vi "MSScript VI Example.vi"() -> ()   [LabVIEW 2018]
uses:
  MSScript.lvclass
panel:
  out "Array":string[](array[string])
  in  "Dialogue":i32(listbox)=-1
  in  "Script of MS Process":string="#Header(IonTrap.R0=10,IonTrap.Z0=7.07106781187,MaxAmp=330);\n$a = 3;\n@Aarr[0:2] = 0 1 2;\n@Barr = 9 8 7 6 5 4 @Aarr @Aarr[0] $a 100;\n#Calc( arradd, @Carr, 3 , $a );\n#Show( @Carr );\n#Show( @Barr );\nSetDAQ:: Channel=0, SampRate=0;\nUpdDO:: Func=1 0 0 0, Val=F F F F;\nUpdAO:: Func=0 0 0 0, Val=0 0 0 0;\n//test2\n//test3\n%\n//test\nPhaseScan:: \n    AuxWfmType=2, AuxStart=30, iAuxCyc=0, AuxCyc=2, Beta=0.5, BetaScale=2, \n    AuxAmp=0, AuxPulse1= 0.40 0.42, AuxPulse2= 0.580 0.60, AuxPulseAmp=1 1,\n    Time = 0.05, Freq=40000 50000, Stepwise=40;\n%\nStop::;\n\n"
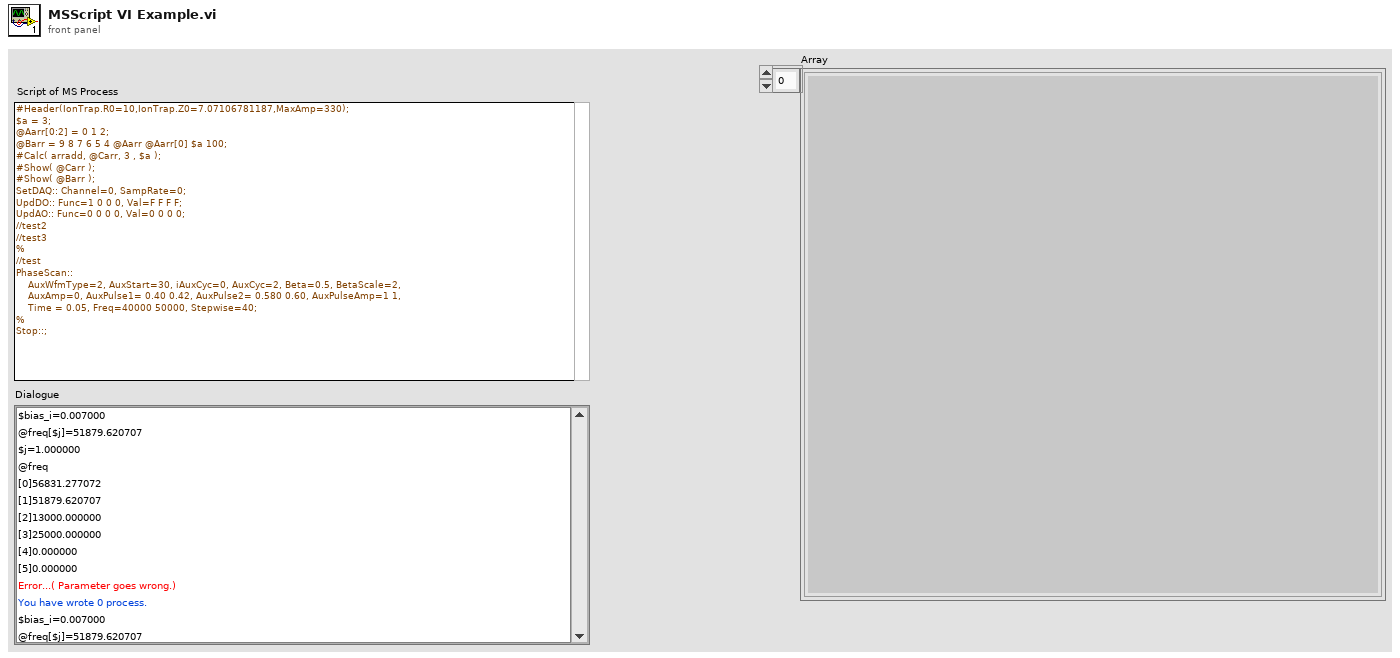
[diagram p1: front panel]
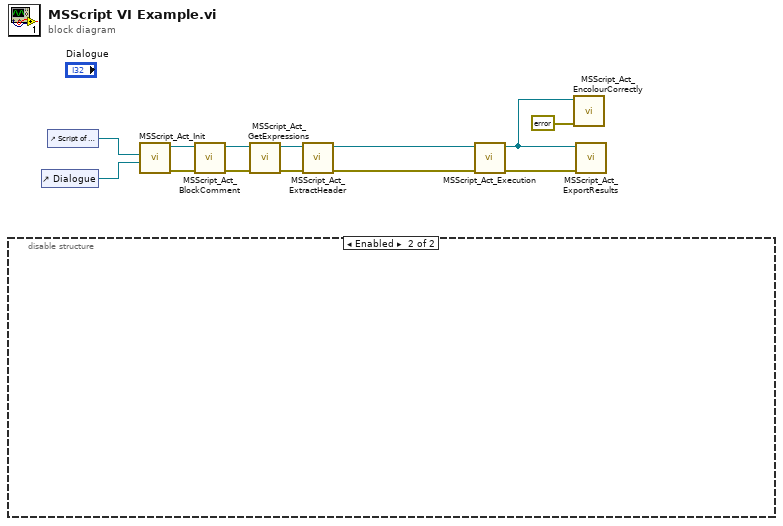
[diagram p0: block diagram]
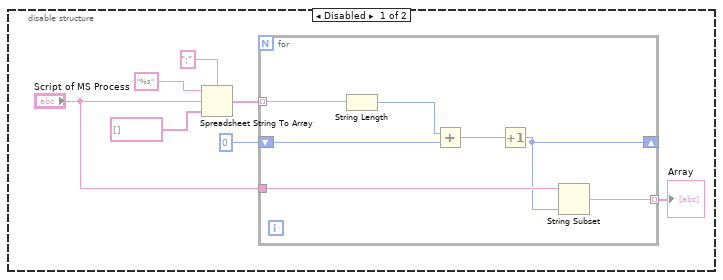
[diagram p2: hidden frame]
diagram:
  n1 = disable-structure shown="Enabled" {
    frame Disabled {
      n2 = Spreadsheet String To Array(delimiter (Tab)=";", format string="%s", spreadsheet string="Script of MS Process", array type (2D Dbl)=string[] []) -> (array=w17:string[])
      n3 = for {
        tunnel: w17 -> [w27] mode=indexing
        shift-right: [w21] -> _
        shift-left: 0 -> [w25]
        tunnel: "Script of MS Process" -> [w24]
        tunnel: [w23] -> w14 mode=indexing
        n4 = String Length(string=w27) -> (length=w26:i32)
        n5 = Add(x=w26, y=w25) -> (x+y=w22:i32)
        n6 = Increment(x=w22) -> (x+1=w21:i32)
        n7 = String Subset(string=w24, length (rest)=w21) -> (substring=w23:string)  [unwired: 1 in]
      }
      "Array" <- w14
    }
    frame Enabled {
    }
  }
  n8 = control-ref of="Dialogue"() -> (w12:refnum<vi>)
  n9 = control-ref of="Script of MS Process"() -> (w13:refnum<vi>)
  n10 = call "MSScript_Act_Init.vi"("Listbox Ref"=w12, "Script ctl ref"=w13) -> ("error out"=w3:errorcluster, "MSScript out"=w4:refnum<class "MSScript.lvclass">)  [unwired: 8 in]
  n11 = call "MSScript_Act_BlockComment.vi"("error in (no error)"=w3, "MSScript in"=w4) -> ("error out"=w1:errorcluster, "MSScript out"=w2:refnum<class "MSScript.lvclass">)  [unwired: 8 in]
  n12 = call-dynamic "MSScript_Act_GetExpressions.vi"("error in (no error)"=w1, "MSScript in"=w2) -> ("error out"=w8:errorcluster, "MSScript out"=w9:refnum<class "MSScript.lvclass">)  [unwired: 8 in]
  n13 = call-dynamic "MSScript_Act_ExtractHeader.vi"("error in (no error)"=w8, "MSScript in"=w9) -> ("error out"=w10:errorcluster, "MSScript out"=w11:refnum<class "MSScript.lvclass">)  [unwired: 8 in]
  n14 = call-dynamic "MSScript_Act_Execution.vi"("error in (no error)"=w10, "MSScript in"=w11) -> ("error out"=w5:errorcluster, "MSScript out"=w6:refnum<class "MSScript.lvclass">)  [unwired: 8 in]
  n15 = call-dynamic "MSScript_Act_EncolourCorrectly.vi"("error in (no error)"=errorcluster {"status"=FALSE, "code"=0, "source"=""}, "MSScript in"=w6) -> ()  [unwired: 8 in, 2 out]
  n16 = call-dynamic "MSScript_Act_ExportResults.vi"("error in (no error)"=w5, "MSScript in"=w6) -> ()  [unwired: 5 in, 5 out]
